vi "Delimiter.vi"() -> (3 "Delimiter":string)   [LabVIEW 2019, in "SLL Environment Variable.lvlib"]
doc: "Assign the delimiter constant <B>(;)</B>"
uses:
  <vilib>/SLL Toolkit/SLL Environment Variable/SLL Environment Variable.lvlib
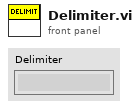
[diagram p1: front panel]
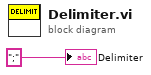
[diagram p0: block diagram]
diagram:
  "Delimiter" <- ";" ("String")
